vi "main OP700.vi"() -> ()   [LabVIEW 2020]
uses:
  SubVI/OP150ZP_state.ctl
  <userlib>/Alex.vi/FGV.ctl
  <vilib>/QMT/GDataBase for MySQL(tm)/MySQL/public/controls/DateType.ctl
  Lib/02 SLIM ZEN WS 500/SubVi/VG_progressBar.vi
  SubVI/CheminDeBase.vi
  <vilib>/Utility/error.llb/Error Cluster From Error Code.vi
  VG/PN.vi
  VG/IS30%.vi
  SubVI/VG_HYDRAU.vi
  VG/VG_BT3562.vi
  <vilib>/QMT/GDataBase for MySQL(tm)/MySQL/MySQLConnector.lvclass
panel:
  out "Revision":i32
  out "error out":errorcluster
  in  "arrêt":bool
  in  "last?":bool
  out "VISA OUT 2":T1
  out "Cluster 2":T2
  out "IS30% ?":bool
  out "BDD":T3
  out "progression":u8(slide) scale=0.0..100.0
  out "PN":string
  out "errout 2":errorcluster={"status"=TRUE, "code"=0, "source"="PCAN_CHANNEL ILLEGAL"} caption="errout"
  out "errout":errorcluster caption="sortie d'erreur"
  out "STOP":bool
  out "TOP":string
  out "DRAW":picture
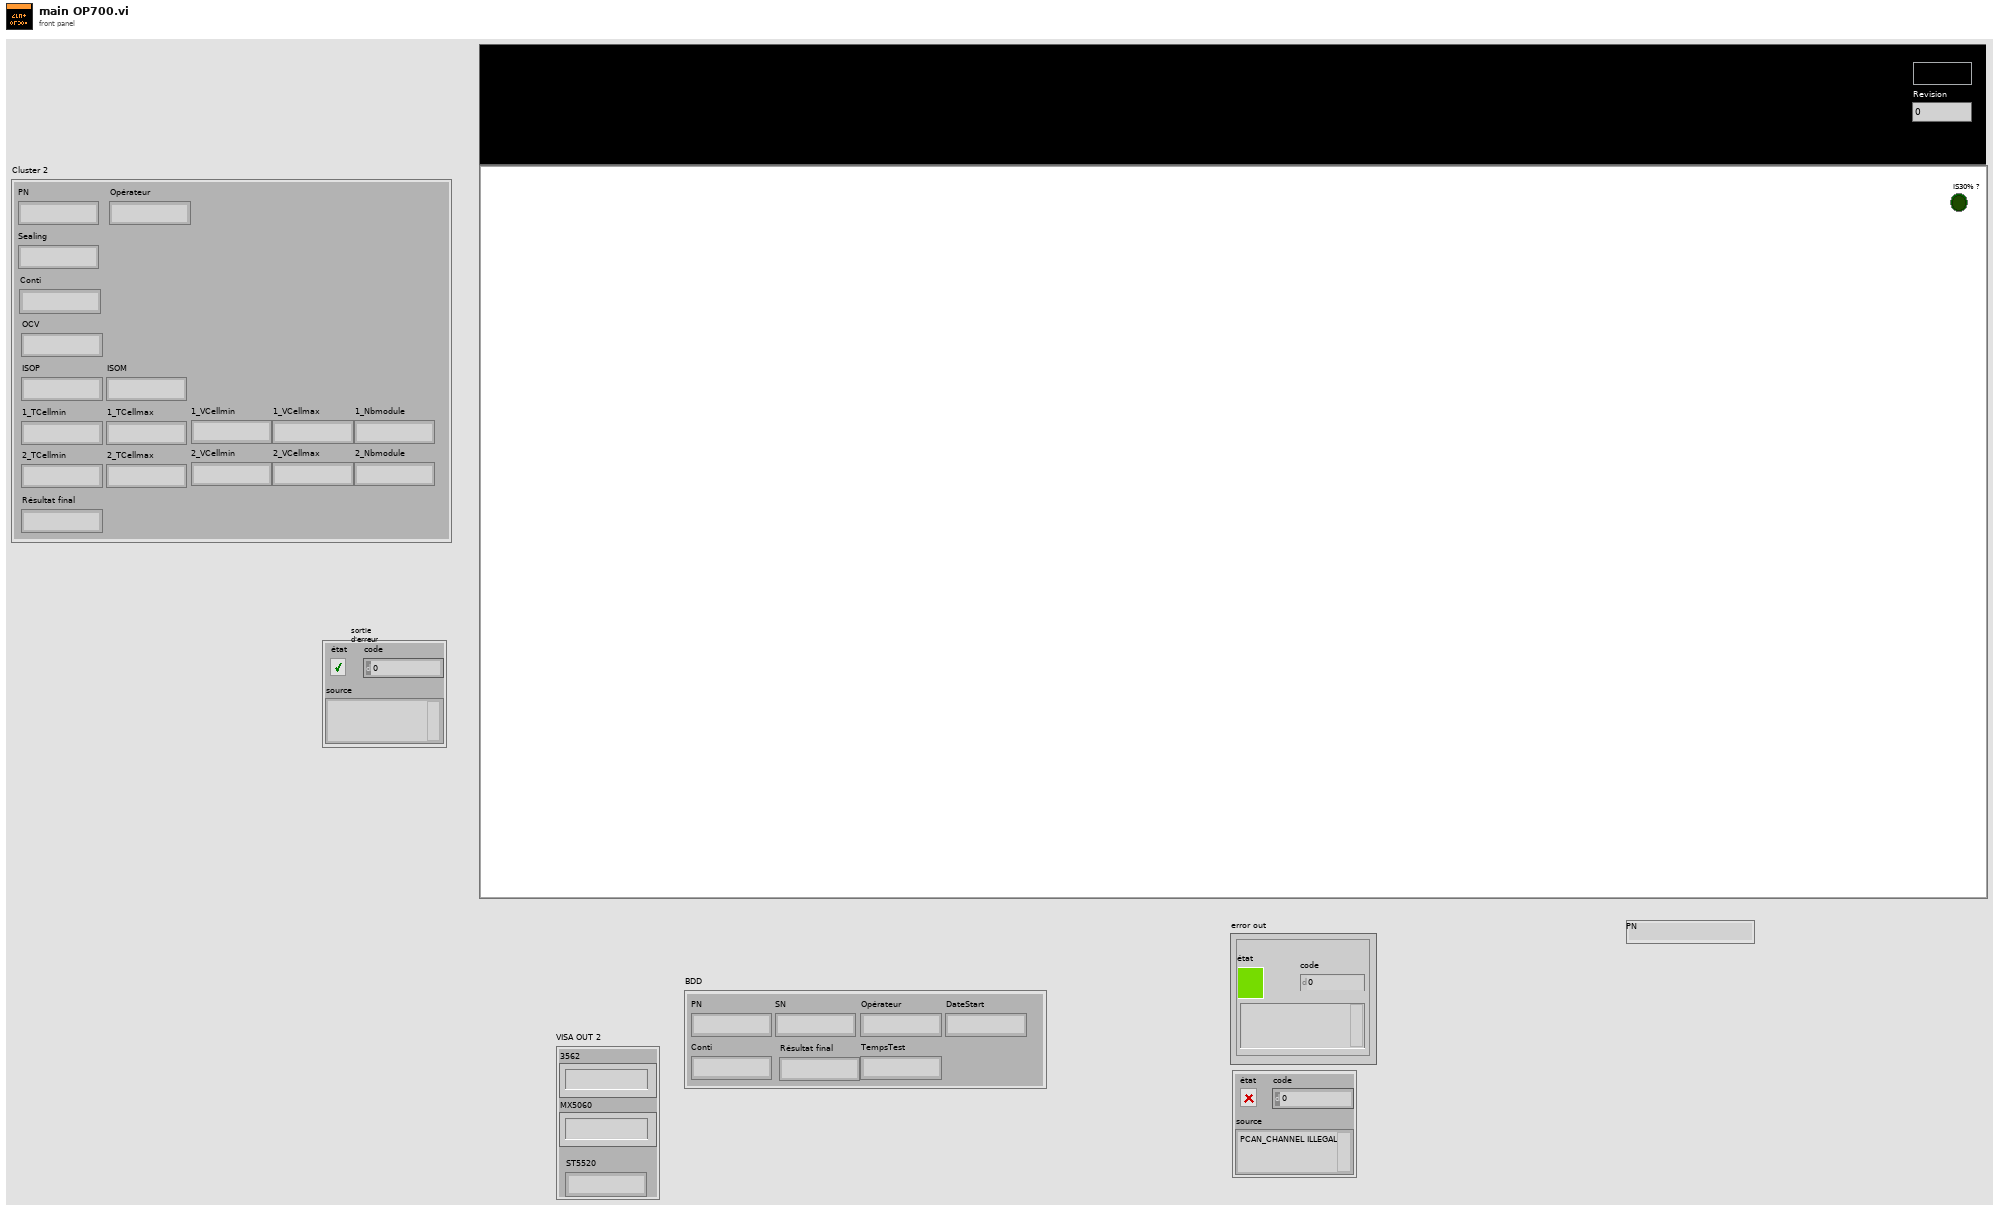
[diagram p1: front panel]
types:
  T1 = cluster{"3562":string, "MX5060":string, "ST5520":string}
  T2 = cluster{"PN":string, "Opérateur":string, "Sealing":string, "Conti":string, "OCV":string, "ISOP":string, "ISOM":string, "1_TCellmin":string, "1_TCellmax":string, "1_VCellmin":string, "1_VCellmax":string, "1_Nbmodule":string, "2_TCellmin":string, "2_TCellmax":string, "2_VCellmin":string, "2_VCellmax":string, "2_Nbmodule":string, "Résultat final":string}
  T3 = cluster{"PN":string, "Opérateur":string, "Conti":string, "Résultat final":string, "SN":string, "DateStart":string, "TempsTest":string}
  T4 = cluster{"PN":string, "Sealing":string, "Opérateur":string, "Conti":string, "OCV":string, "ISOP":string, "ISOP 2":string}
  T5 = typedef "OP150ZP_state.ctl" = enum16{"Null", "Demarrage", "Init", "Scan", "Crash", "Next", "Conti", "Sealing", "Comext", ""}
  T6 = typedef "FGV.ctl" = enum16{"GET", "SET", "RAZ"}
  T7 = typedef "MySQLVIEW.lvlib/MySQLConnector.lvclass/DateType.ctl" = enum16{"DATETIME", "DATE", "TIMESTAMP", "TIME", "YEAR (2 digits)", "YEAR (4 digits)"}
  T8 = typedef "imagedata.ctl" = cluster{"image type":i32, "image depth":i32, "image":u8[], "mask":u8[], "colors":u32[], "Rectangle":cluster{"left":i16, "top":i16, "right":i16, "bottom":i16}}
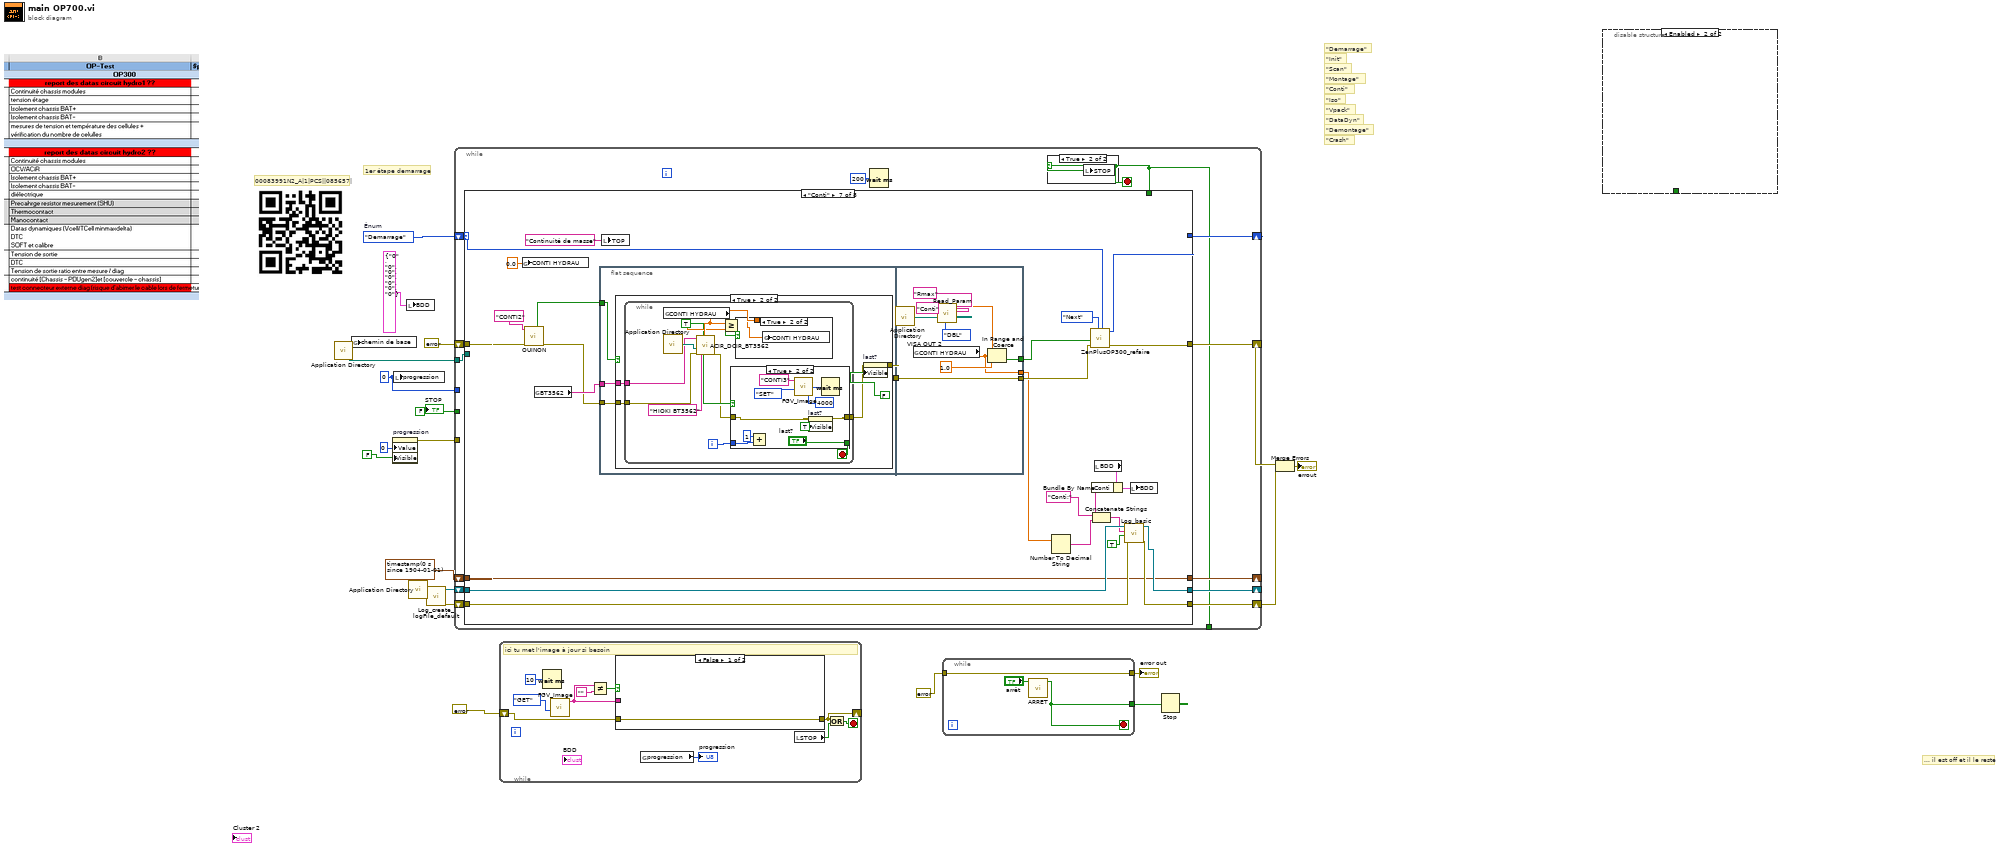
[diagram p0: block diagram]
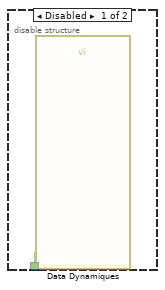
[diagram p2: hidden frame]
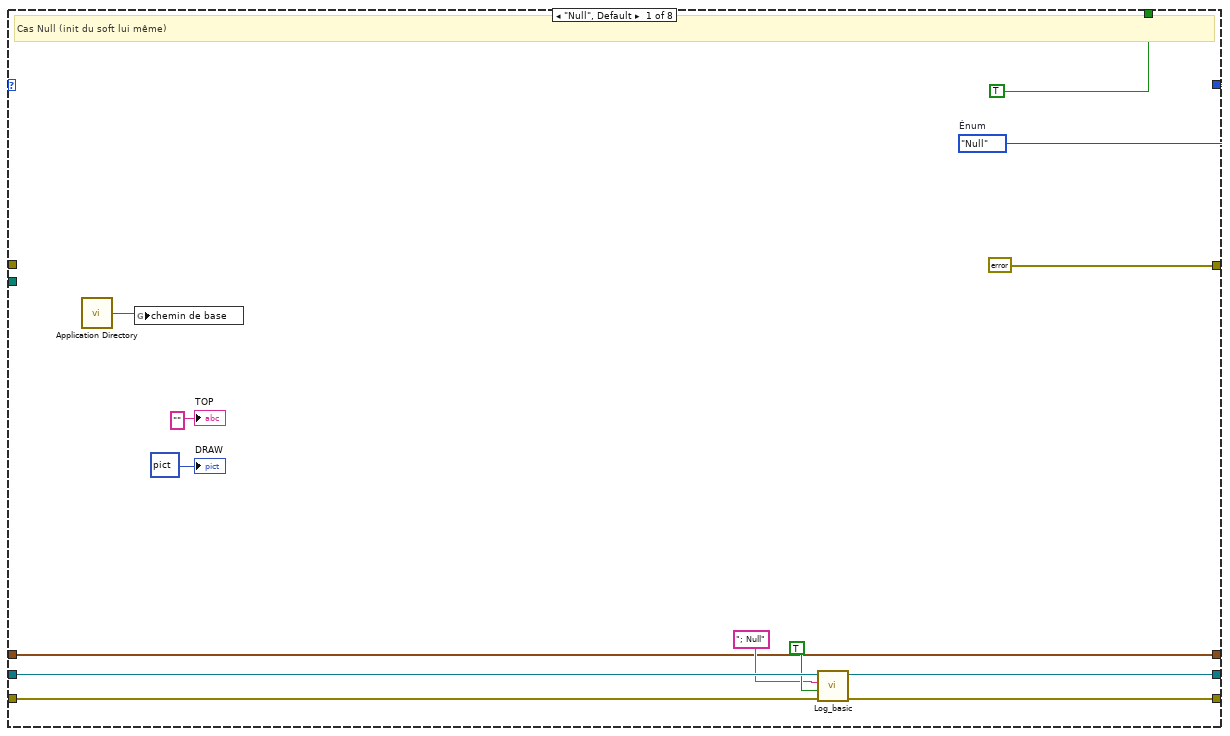
[diagram p4: hidden frame]
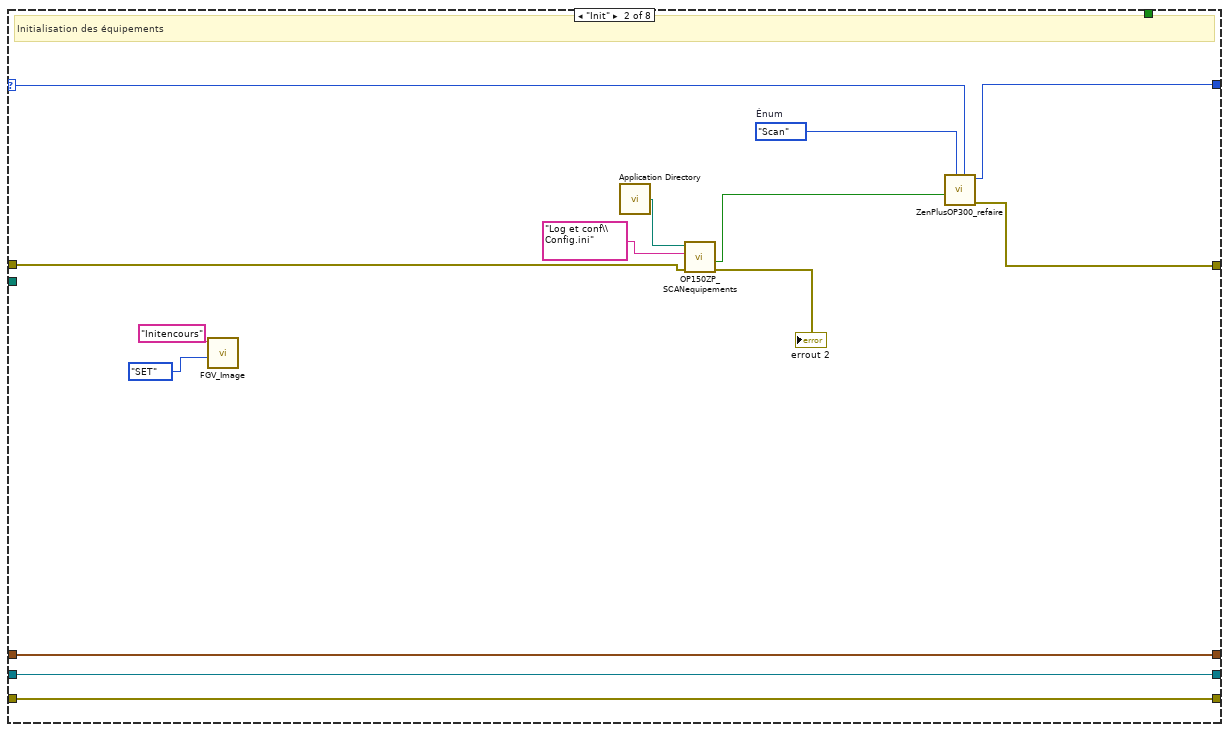
[diagram p5: hidden frame]
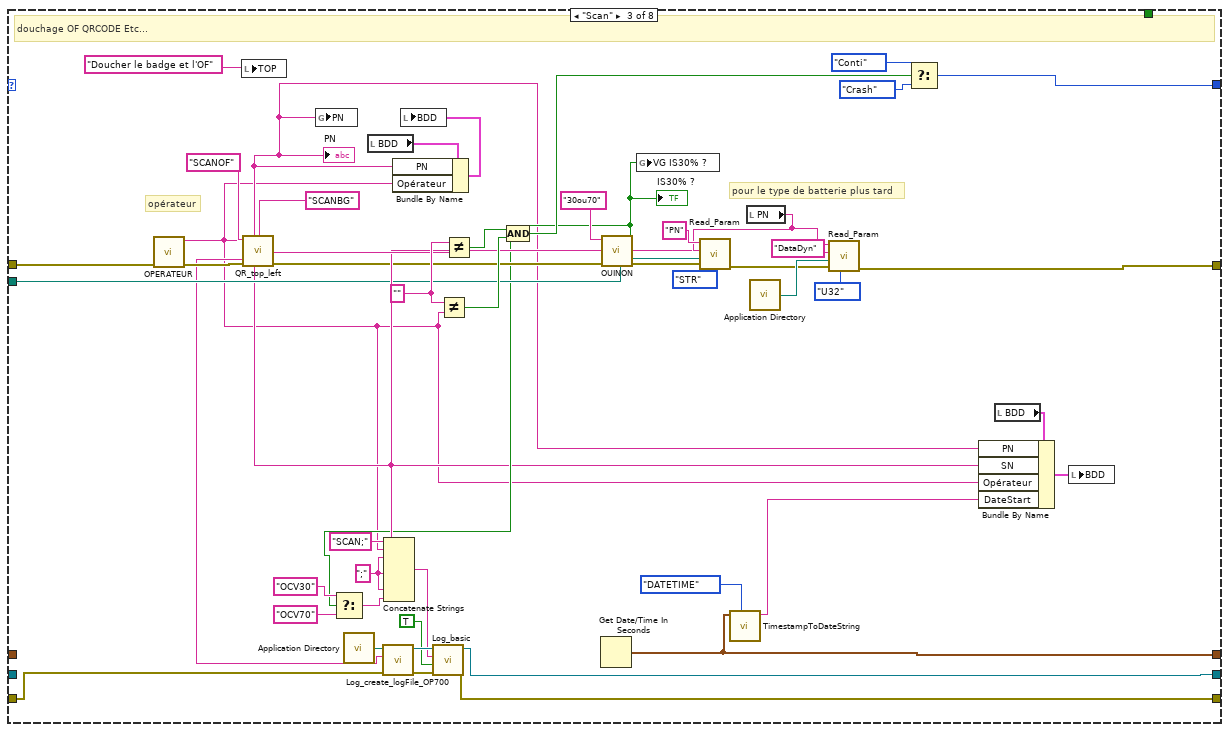
[diagram p6: hidden frame]
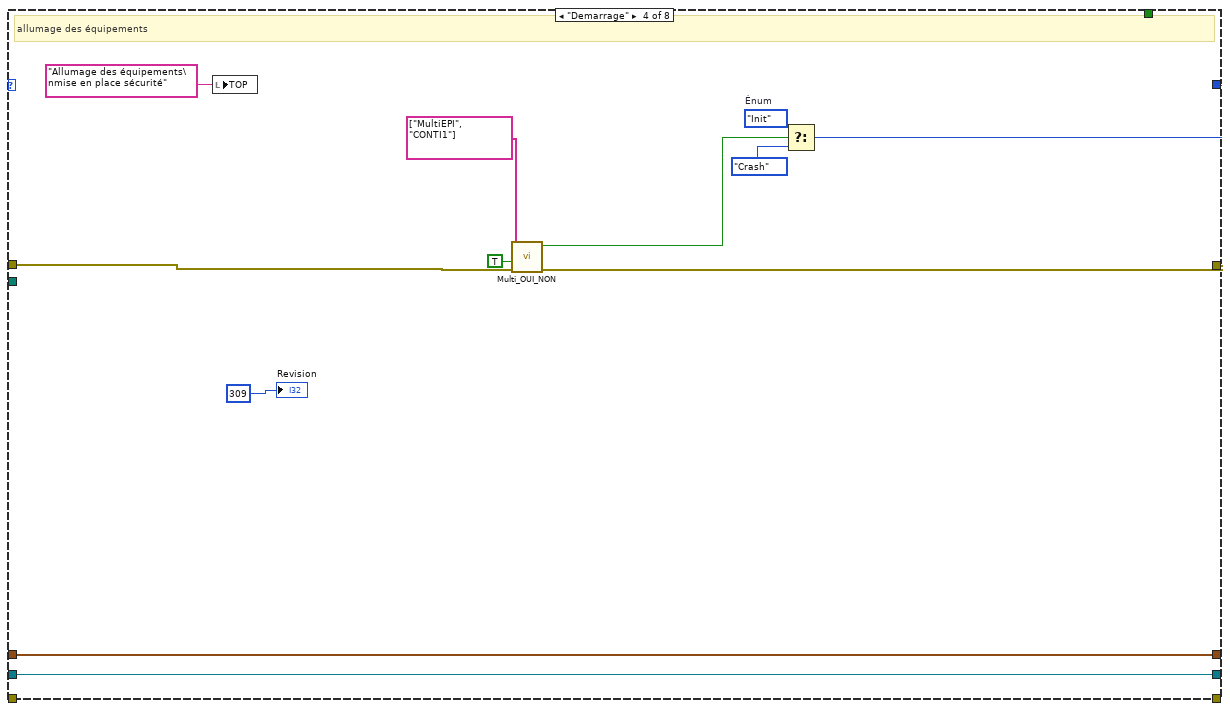
[diagram p7: hidden frame]
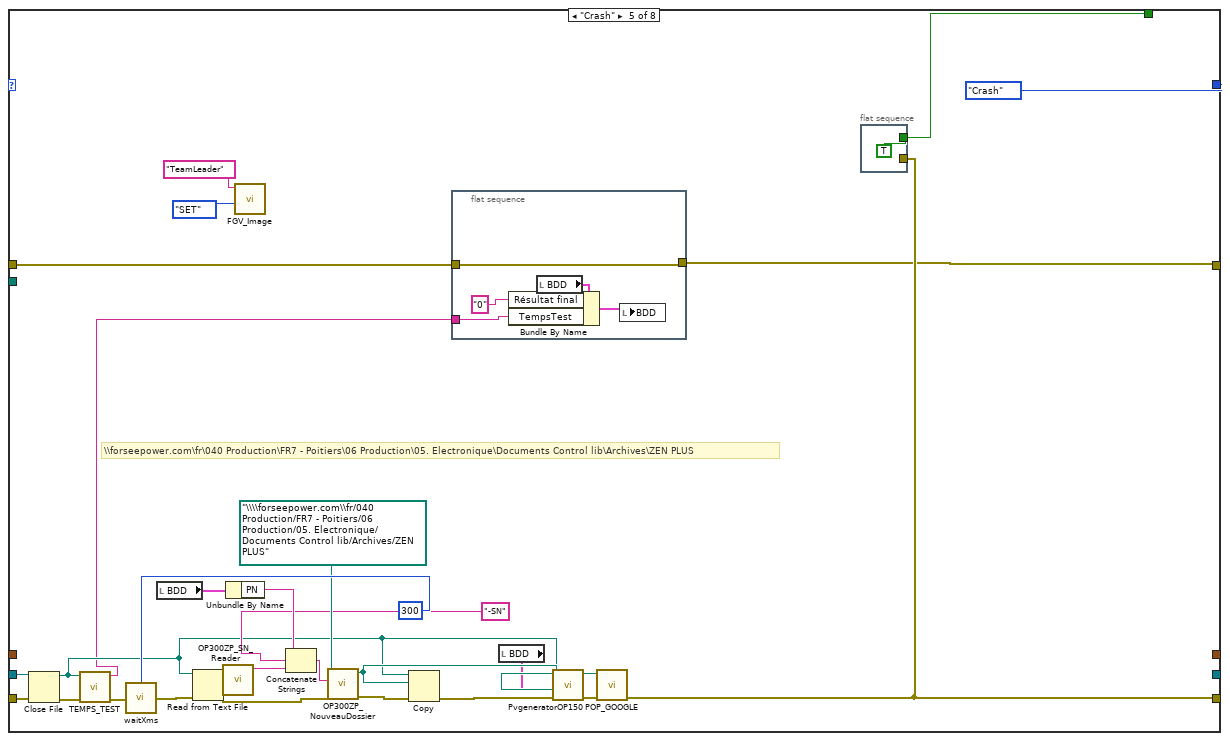
[diagram p8: hidden frame]
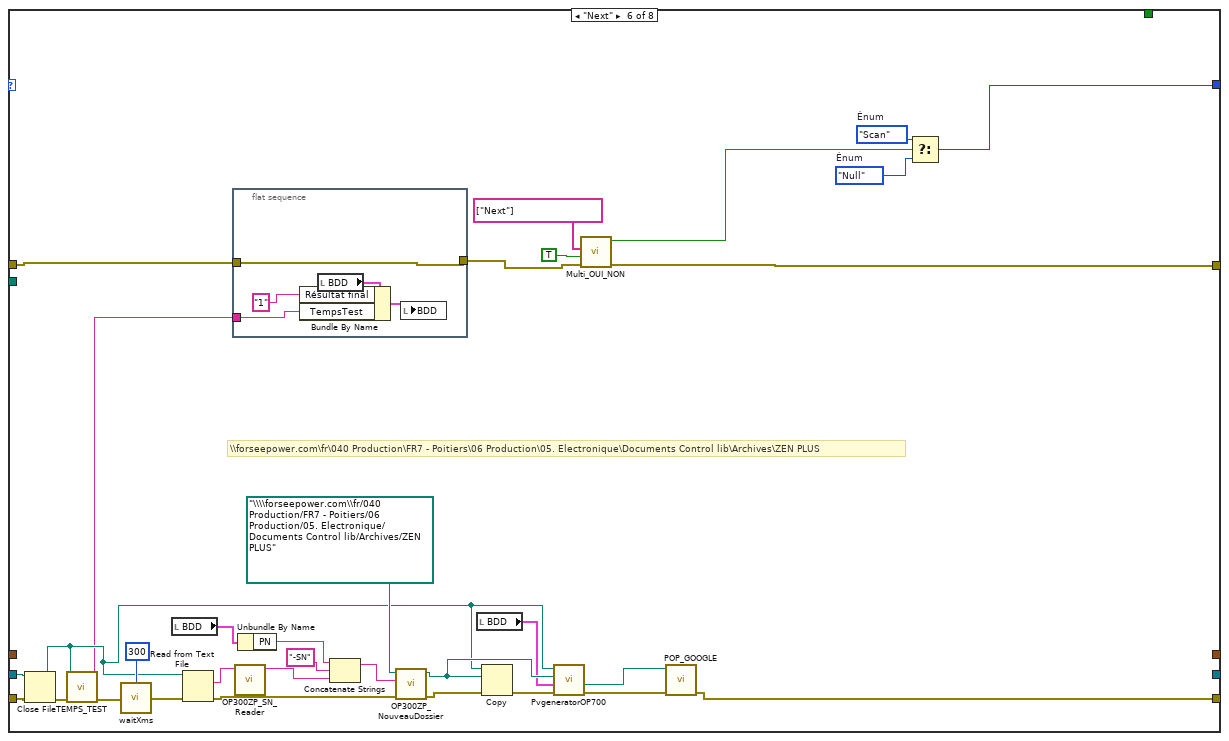
[diagram p9: hidden frame]
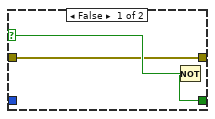
[diagram p11: hidden frame]
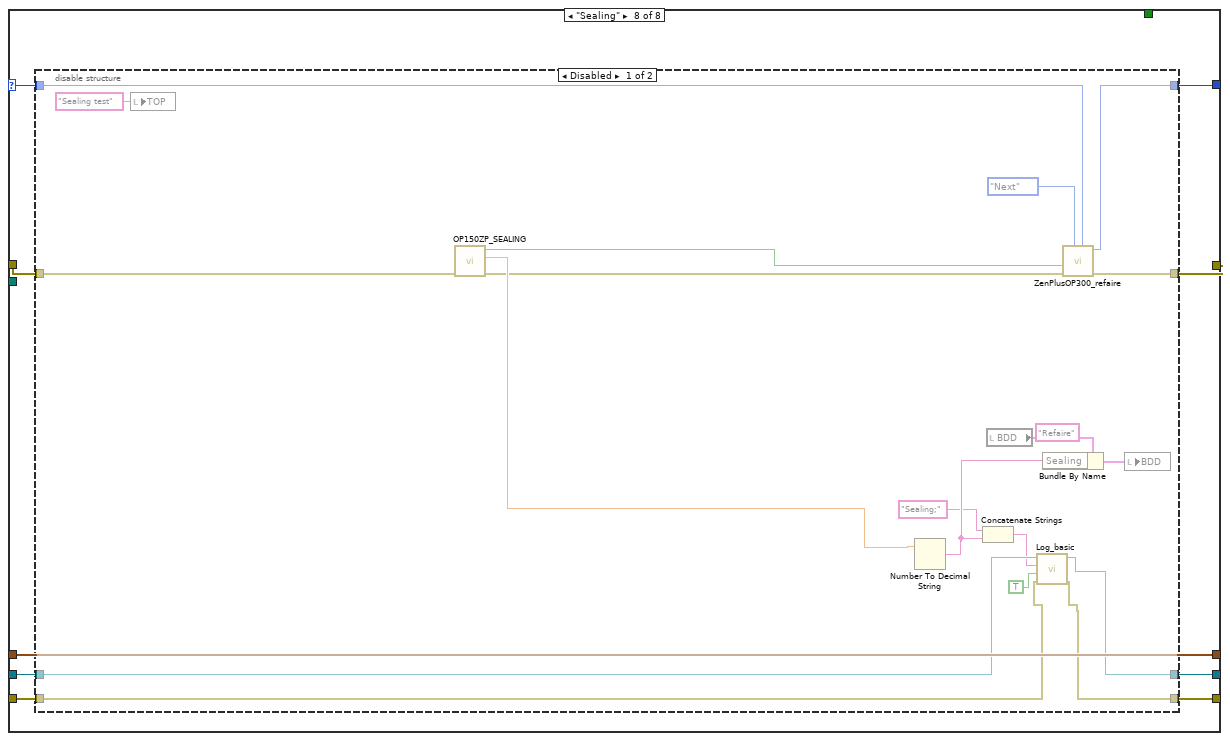
[diagram p13: hidden frame]
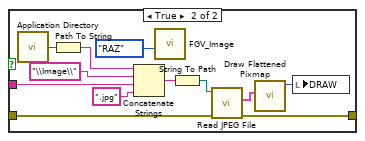
[diagram p15: hidden frame]
diagram:
  w10 = u8 0 ("progression")
  w11 = OP150ZP_state."Demarrage"  # Énum
  w17 = FALSE ("STOP")
  # "00083991N2_A|1|PCS||085657|"
  # "1er étape demarrage"
  # "\"Crash\""
  # "\"Demontage\""
  # "\"DataDyn\""
  # "\"Iso\""
  # "\"Montage\""
  # "\"Scan\""
  # "\"Init\""
  # "\"Demarrage\""
  # "\"Conti\""
  # "\"Vpack\""
  # "... il est off et il le reste"
  n1 = call <vilib>:"Application Directory.vi"() -> ("Application Directory"=w16:path)
  n2 = global write "CheminDeBase.vi" "chemin de base"(w16) -> ()
  n3 = property on="progression" class="Slide (strict)"("Value"=u8 0 ("progression"), "Visible"=FALSE) -> (error out=w8:errorcluster)  [unwired: 2 in, 1 out]
  n4 = local write "progression"(w10) -> ()
  n5 = local write "BDD"(T4 {"PN"="0", "Sealing"="0", "Opérateur"="0", "Conti"="0", "OCV"="0", "ISOP"="0", "ISOP 2"="0"} ("Cluster")) -> ()
  n6 = call <vilib>:"Application Directory.vi"() -> ("Application Directory"=w14:path)
  n7 = call "Log_create_logFile_default.vi"("appdir"=w14) -> ("errout"=w15:errorcluster, "Fichier à flux d'octets en sortie"=w18:refnum<file>)  [unwired: 9 in]
  n8 = while {
    shift-right: [w32] -> w3
    shift-left: errorcluster {"status"=FALSE, "code"=0, "source"=""} ("error out") -> [w23]
    shift-right: [w22] -> _
    shift-left: w11 -> [w27]
    shift-right: [w28] -> w19
    shift-left: w15 -> [w31]
    shift-right: [w29] -> _
    shift-left: w18 -> [w30]
    tunnel: w16 -> [w26]
    tunnel: w17 -> [_]
    shift-right: [w24] -> _
    shift-left: timestamp(0 s since 1904-01-01) ("seconds since 1Jan1904") -> [w25]
    tunnel: w10 -> [_]
    tunnel: w8 -> [_]
    tunnel: [w21] -> _
    stop <- w21 stop-if-true
    n9 = case shown="\"Conti\"" w27 {
      selector: w27 -> [_ w56 _ _ _ _ w220 w268]
      tunnel: w23 -> [_ w58 w111 w115 w129 w166 w221 w267]
      tunnel: [errorcluster {"status"=FALSE, "code"=0, "source"=""} ("errin") w57 w92 w122 w128 w170 w213 w272] -> w32
      tunnel: w31 -> [w43 w61 w107 _ w150 w189 w218 w275]
      tunnel: w30 -> [w44 w60 _ w123 w151 w190 w216 w274]
      tunnel: [w41 w60 w109 w123 _ _ w215 w273] -> w29
      tunnel: [w42 w61 w110 _ w142 w183 w217 w270] -> w28
      tunnel: [TRUE _ _ _ w152 _ _ _] -> w21
      tunnel: w26 -> [_ _ w86 _ _ _ _ _]
      tunnel: w25 -> [w37 w59 _ w121 _ _ w214 w271]
      tunnel: [w37 w59 w65 w121 _ _ w214 w271] -> w24
      tunnel: [w35 w48 w70 w116 OP150ZP_state."Crash" w167 w219 w269] -> w22
      frame "Null", Default {
        w35 = OP150ZP_state."Null"  # Énum
        # "Cas Null (init du soft lui même)"
        n10 = call <vilib>:"Application Directory.vi"() -> ("Application Directory"=w47:path)
        n11 = global write "CheminDeBase.vi" "chemin de base"(w47) -> ()
        n12 = call "Log_basic.vi"("errin"=w43, "date?"=TRUE, "chaîne"="; Null", "in"=w44) -> ("sortie d'erreur"=w42:errorcluster, "refnum en sortie"=w41:refnum<file>)  [unwired: 6 in]
        "DRAW" <- picture data[5B] ("DRAW")
        "TOP" <- "" ("TOP")
      }
      frame "Init" {
        w52 = OP150ZP_state."Scan"  # Énum
        # "Initialisation des équipements"
        n13 = call <userlib>:"FGV_Image.vi"("Énum"=FGV."SET", "IN"="Initencours") -> ()  [unwired: 9 in, 1 out]
        n14 = call <vilib>:"Application Directory.vi"() -> ("Application Directory"=w49:path)
        n15 = call "OP150ZP_SCANequipements.vi"("Errin"=w58, "Chaîne"="Log et conf\\Config.ini", "pathin"=w49) -> ("ERROUT"=→"errout 2":errorcluster, "KO?"=w53:bool)  [unwired: 7 in]
        n16 = call "ZenPlusOP300_refaire.vi"("refaire"=w56, "casOK"=w52, "test ok ?"=w53) -> ("errout"=w57:errorcluster, "Next"=w48:T5)  [unwired: 7 in]
      }
      frame "Scan" {
        w73 = ";" ("chaîne")
        w101 = "" ("x")
        # "pour le type de batterie plus tard"
        # "opérateur"
        # "douchage OF QRCODE Etc..."
        n17 = call "OPERATEUR.vi"("errin"=w111, "IN"="SCANBG") -> ("error out"=w98:errorcluster, "Dataout"=w66:string)  [unwired: 8 in]
        n18 = local write "TOP"("Doucher le badge et l'OF" ("TOP")) -> ()
        n19 = call "QR_top_left.vi"("errin"=w98, "image"="SCANOF") -> ("error out"=w77:errorcluster, "Réponse"=w96:string, "SN"=w67:string, "PN"=w68:string)  [unwired: 5 in, 1 out]
        "PN" <- w68
        n20 = global write "PN.vi" "PN"(w68) -> ()
        n21 = call <vilib>:"Application Directory.vi"() -> ("Application Directory"=w108:path)
        n22 = local read "BDD"() -> (w80:T3)
        n23 = call "Log_create_logFile_OP700.vi"("errin"=w107, "toute l'expression"=w67, "Application Directory"=w108) -> ("sortie d'erreur"=w105:errorcluster, "Fichier à flux d'octets en sortie"=w106:refnum<file>)  [unwired: 7 in]
        n24 = Bundle By Name(cluster=w80, "PN"=w68, "Opérateur"=w66) -> (w79:T3)
        n25 = local write "BDD"(w79) -> ()
        n26 = Not Equal?(x=w101, y=w66) -> (x != y?=w99:bool)
        n27 = Not Equal?(x=w101, y=w96) -> (x != y?=w100:bool)
        n28 = Compound Arithmetic op=AND ("Opérateur arithmétique")(w100, w99) -> (w84:bool)
        n29 = Get Date/Time In Seconds() -> (seconds since 1Jan1904=w65:timestamp)
        n30 = call "OUINON.vi"("errin"=w77, "image"="30ou70") -> ("error out"=w76:errorcluster, "OUI/NON"=w71:bool)  [unwired: 8 in]
        "IS30% ?" <- w71
        n31 = Select ("Sélectionner")(t="OCV30" ("section"), s=w71, f="OCV70" ("section")) -> (s? t:f=w72:string)
        n32 = global write "IS30%.vi" "VG IS30% ?"(w71) -> ()
        n33 = call <vilib>:"TimestampToDateString.vi"("dateType"=DateType."DATETIME", "timestamp in"=w65) -> ("dateString"=w64:string)  [unwired: 8 in, 1 out]
        n34 = local read "PN"() -> (w88:string)
        n35 = call "Read_Param.vi"("Énum"=enum16{"STR", "DBL", "U32"}."STR", "errin"=w76, "pathin"=w86, "section"=w88, "key"="PN") -> ("error out"=w91:errorcluster, "str"=w87:string)  [unwired: 2 in, 3 out]
        n36 = Concatenate Strings("SCAN;" ("chaîne"), w66, w73, w67, w73, w87, w73, w72) -> (w103:string)
        n37 = call "Log_basic.vi"("errin"=w105, "date?"=TRUE, "chaîne"=w103, "in"=w106) -> ("sortie d'erreur"=w110:errorcluster, "refnum en sortie"=w109:refnum<file>)  [unwired: 6 in]
        n38 = call <vilib>:"Application Directory.vi"() -> ("Application Directory"=w95:path)
        n39 = call "Read_Param.vi"("Énum"=enum16{"STR", "DBL", "U32"}."U32", "errin"=w91, "pathin"=w95, "section"="DataDyn", "key"=w88) -> ("error out"=w92:errorcluster)  [unwired: 2 in, 4 out]
        n40 = Select ("Sélectionner")(t=OP150ZP_state."Conti" ("Énum"), s=w84, f=OP150ZP_state."Crash" ("cas faux")) -> (s? t:f=w70:T5)
        n41 = local read "BDD"() -> (w69:T3)
        n42 = Bundle By Name(cluster=w69, "PN"=w68, "SN"=w67, "Opérateur"=w66, "DateStart"=w64) -> (w63:T3)
        n43 = local write "BDD"(w63) -> ()
      }
      frame "Demarrage" {
        w118 = OP150ZP_state."Init"  # Énum
        # "allumage des équipements"
        n44 = local write "TOP"("Allumage des équipements\nmise en place sécurité" ("TOP")) -> ()
        n45 = call "Multi_OUI_NON.vi"("errin"=w115, "errinb"=TRUE, "Tableau"=string[] ["MultiEPI", "CONTI1"]) -> ("errout"=w122:errorcluster, "isok?"=w119:bool)  [unwired: 7 in]
        n46 = Select ("Sélectionner")(t=w118, s=w119, f=OP150ZP_state."Crash" ("cas faux")) -> (s? t:f=w116:T5)
        "Revision" <- 309
      }
      frame "Crash" {
        # "\\\\forseepower.com\\fr\\040 Production\\FR7 - Poitiers\\06 Production\\05. Electronique\\Documents Control lib\\Archives\\ZEN PLUS"
        n47 = Close File(refnum=w151, error in=w150) -> (path=w126:path, error out=w144:errorcluster)
        n48 = call <userlib>:"TEMPS_TEST.vi"("errin"=w144, "pathin"=w126) -> ("error out"=w127:errorcluster, "Delay calculé"=w125:string)  [unwired: 8 in]
        n49 = call <userlib>:"waitXms.vi"("attente (ms)"=u32 300, "errin"=w127) -> ("errout"=w141:errorcluster)  [unwired: 13 in]
        n50 = local read "BDD"() -> (w135:T3)
        n51 = Read from Text File(file (use dialog)=w126, error in=w141) -> (text=w140:string, error out=w138:errorcluster)  [unwired: 2 in, 2 out]
        n52 = call "OP300ZP_SN_Reader.vi"("Fichier txt"=w140) -> ("SN"=w133:string)  [unwired: 10 in]
        n53 = Unbundle By Name(w135) -> ("PN"=w132:string)
        n54 = call <userlib>:"FGV_Image.vi"("Énum"=FGV."SET", "IN"="TeamLeader") -> ()  [unwired: 9 in, 1 out]
        n55 = Concatenate Strings(w132, "-SN" ("chaîne"), w133) -> (w134:string)
        n56 = call "OP300ZP_NouveauDossier.vi"("entrée d'erreur (pas d'erreur)"=w138, "Nom du repertoire (PN SN)"=w134, "Network before adding a new folder"=path "\\\\forseepower.com\\fr/040 Production/FR7 - Poitiers/06 Production/05. Electronique/Documents Control lib/Archives/ZEN PLUS" ("chemin de la cible (utiliser une boîte de dialogue)")) -> ("sortie d'erreur"=w139:errorcluster, "Network after adding a new folder"=w136:path)  [unwired: 7 in]
        n57 = Copy ("Copier")(8:w139, 10:w136, 11:w126) -> (0:w143:errorcluster)  [unwired: 2 in, 2 out]
        n58 = flat-sequence {
          tunnel: [w155] -> w128
          tunnel: w129 -> [w155]
          tunnel: w125 -> [w153]
          frame #0 {
            n59 = local read "BDD"() -> (w157:T3)
            n60 = Bundle By Name(cluster=w157, "Résultat final"="0", "TempsTest"=w153) -> (w154:T3)
            n61 = local write "BDD"(w154) -> ()
          }
        }
        n62 = local read "BDD"() -> (w124:T3)
        n63 = call "PvgeneratorOP150.vi"("errin"=w143, "BDD"=w124, "network"=w136, "path in"=w126) -> ("sortie d'erreur"=w147:errorcluster, "network out"=w146:path)  [unwired: 4 in, 2 out]
        n64 = call "POP_GOOGLE.vi"("error in"=w147, "chemin"=w146) -> ("error out"=w142:errorcluster)  [unwired: 8 in, 1 out]
        n65 = flat-sequence {
          tunnel: [TRUE] -> w152
          tunnel: w142 -> [_]
          frame #0 {
          }
        }
      }
      frame "Next" {
        w187 = OP150ZP_state."Null"  # Énum
        w188 = OP150ZP_state."Scan"  # Énum
        # "\\\\forseepower.com\\fr\\040 Production\\FR7 - Poitiers\\06 Production\\05. Electronique\\Documents Control lib\\Archives\\ZEN PLUS"
        n66 = Close File(refnum=w190, error in=w189) -> (path=w163:path, error out=w164:errorcluster)
        n67 = call <userlib>:"TEMPS_TEST.vi"("errin"=w164, "pathin"=w163) -> ("error out"=w161:errorcluster, "Delay calculé"=w160:string)  [unwired: 8 in]
        n68 = call <userlib>:"waitXms.vi"("attente (ms)"=u32 300, "errin"=w161) -> ("errout"=w162:errorcluster)  [unwired: 13 in]
        n69 = local read "BDD"() -> (w176:T3)
        n70 = Read from Text File(file (use dialog)=w163, error in=w162) -> (text=w181:string, error out=w180:errorcluster)  [unwired: 2 in, 2 out]
        n71 = flat-sequence {
          tunnel: [w193] -> w165
          tunnel: w166 -> [w193]
          tunnel: w160 -> [w191]
          frame #0 {
            n72 = local read "BDD"() -> (w195:T3)
            n73 = Bundle By Name(cluster=w195, "Résultat final"="1", "TempsTest"=w191) -> (w192:T3)
            n74 = local write "BDD"(w192) -> ()
          }
        }
        n75 = call "OP300ZP_SN_Reader.vi"("Fichier txt"=w181) -> ("SN"=w173:string)  [unwired: 10 in]
        n76 = Unbundle By Name(w176) -> ("PN"=w175:string)
        n77 = Concatenate Strings(w175, "-SN" ("chaîne"), w173) -> (w172:string)
        n78 = call "OP300ZP_NouveauDossier.vi"("entrée d'erreur (pas d'erreur)"=w180, "Nom du repertoire (PN SN)"=w172, "Network before adding a new folder"=path "\\\\forseepower.com\\fr/040 Production/FR7 - Poitiers/06 Production/05. Electronique/Documents Control lib/Archives/ZEN PLUS" ("chemin de la cible (utiliser une boîte de dialogue)")) -> ("sortie d'erreur"=w179:errorcluster, "Network after adding a new folder"=w177:path)  [unwired: 7 in]
        n79 = local read "BDD"() -> (w159:T3)
        n80 = Copy ("Copier")(8:w179, 10:w177, 11:w163) -> (0:w182:errorcluster)  [unwired: 2 in, 2 out]
        n81 = call "PvgeneratorOP700.vi"("errin"=w182, "BDD"=w159, "network"=w177, "path in"=w163) -> ("sortie d'erreur"=w185:errorcluster, "network out"=w184:path)  [unwired: 4 in, 2 out]
        n82 = call "Multi_OUI_NON.vi"("errin"=w165, "errinb"=TRUE, "Tableau"=string[] ["Next"]) -> ("errout"=w170:errorcluster, "isok?"=w169:bool)  [unwired: 7 in]
        n83 = call "POP_GOOGLE.vi"("error in"=w185, "chemin"=w184) -> ("error out"=w183:errorcluster)  [unwired: 8 in, 1 out]
        n84 = Select(t=w188, s=w169, f=w187) -> (s? t:f=w167:T5)
      }
      frame "Conti" {
        n85 = global write "VG_HYDRAU.vi" "CONTI HYDRAU"(0.0 ("R")) -> ()
        n86 = call "OUINON.vi"("errin"=w221, "image"="CONTI2" ("IN")) -> ("error out"=w196:errorcluster, "OUI/NON"=w208:bool)  [unwired: 8 in]
        n87 = global read "VG_BT3562.vi" "BT3562"() -> (w203:string)
        n88 = flat-sequence {
          tunnel: w208 -> [w225]
          tunnel: w203 -> [w224]
          tunnel: [w223] -> w212
          tunnel: w196 -> [w222]
          tunnel: [w260] -> w204
          tunnel: [w259] -> w205
          tunnel: [w258] -> w206
          tunnel: w212 -> [w258]
          frame #0 {
            n89 = case shown="True" w225 {
              tunnel: w224 -> [_ w231]
              tunnel: [w226 w229] -> w223
              tunnel: w222 -> [w226 w227]
              frame False {
              }
              frame True {
                n90 = while {
                  tunnel: w231 -> [w235]
                  tunnel: [w242] -> w228
                  tunnel: w227 -> [w233]
                  i -> [w241]
                  stop <- w238 stop-if-true
                  n91 = global read "VG_HYDRAU.vi" "CONTI HYDRAU"() -> (w236:dbl)
                  n92 = call <vilib>:"Application Directory.vi"() -> ("Application Directory"=w244:path)
                  n93 = call <userlib>:"ACIR_DCIR_BT3562.vi"("juste R?"=TRUE, "errin"=w233, "chemin de base"=w244, "section"="HIOKI BT3562", "VISAin"=w235) -> ("errout"=w237:errorcluster, "OK?"=w243:bool, "R"=w239:dbl)  [unwired: 4 out]
                  n94 = Greater Or Equal?(x=w239, y=w236) -> (x >= y?=w240:bool)
                  n95 = case shown="True" w243 {
                    selector: w243 -> [w247 _]
                    tunnel: w237 -> [w245 w249]
                    tunnel: [w245 w251] -> w242
                    tunnel: [w246 "last?"] -> w238
                    tunnel: w241 -> [_ w254]
                    frame False {
                      n96 = Not(x=w247) -> (.not. x?=w246:bool)
                    }
                    frame True {
                      n97 = Add(x=1, y=w254) -> ()  [unwired: 1 out]
                      n98 = call <userlib>:"FGV_Image.vi"("Énum"=FGV."SET", "IN"="CONTI3") -> ()  [unwired: 9 in, 1 out]
                      n99 = property on="last?" class="Bool"(error in=w249, "Visible"=TRUE) -> (error out=w251:errorcluster)  [unwired: 1 in, 1 out]
                      n100 = Wait (ms)(milliseconds to wait=u32 4000 ("attente (ms)")) -> ()  [unwired: 1 out]
                    }
                  }
                  n101 = case shown="True" w240 {
                    tunnel: w239 -> [_ w257]
                    frame False {
                    }
                    frame True {
                      n102 = global write "VG_HYDRAU.vi" "CONTI HYDRAU"(w257) -> ()
                    }
                  }
                }
                n103 = property on="last?" class="Bool"(error in=w228, "Visible"=FALSE) -> (error out=w229:errorcluster)  [unwired: 1 in, 1 out]
              }
            }
          }
          frame #1 {
            n104 = call <vilib>:"Application Directory.vi"() -> ("Application Directory"=w264:path)
            n105 = global read "VG_HYDRAU.vi" "CONTI HYDRAU"() -> (w259:dbl)
            n106 = call "Read_Param.vi"("Énum"=enum16{"STR", "DBL", "U32"}."DBL", "pathin"=w264, "section"="Conti", "key"="Rmax") -> ("dbl"=w262:dbl)  [unwired: 3 in, 4 out]
            n107 = In Range and Coerce(upper limit=w262, x=w259, lower limit=1.0 ("limite inférieure")) -> (In Range?=w260:bool)  [unwired: 1 out]
          }
        }
        n108 = local write "TOP"("Continuité de masse" ("TOP")) -> ()
        n109 = Number To Decimal String(number=w205) -> (decimal integer string=w200:string)  [unwired: 1 in]
        n110 = call "ZenPlusOP300_refaire.vi"("refaire"=w220, "casOK"=OP150ZP_state."Next" ("refaire"), "errin"=w206, "test ok ?"=w204) -> ("errout"=w213:errorcluster, "Next"=w219:T5)  [unwired: 6 in]
        n111 = Concatenate Strings("Conti;" ("chaîne"), w200) -> (w198:string)
        n112 = local read "BDD"() -> (w201:T3)
        n113 = Bundle By Name(cluster=w201, "Conti"=w200) -> (w202:T3)
        n114 = call "Log_basic.vi"("errin"=w218, "date?"=TRUE, "chaîne"=w198, "in"=w216) -> ("sortie d'erreur"=w217:errorcluster, "refnum en sortie"=w215:refnum<file>)  [unwired: 6 in]
        n115 = local write "BDD"(w202) -> ()
      }
      frame "Sealing" {
        n116 = disable-structure shown="Disabled" {
          disable-tunnel: w275 -> [w294 _]
          disable-tunnel: w274 -> [w293 _]
          disable-tunnel: [w292 _] -> w273
          disable-tunnel: [w291 _] -> w272
          disable-tunnel: [w287 _] -> w270
          disable-tunnel: [w286 _] -> w269
          disable-tunnel: w268 -> [w284 _]
          disable-tunnel: w267 -> [w282 _]
          frame Disabled {
            (unwired) "Refaire" ("image")
            n117 = local write "TOP"("Sealing test" ("TOP")) -> ()
            n118 = call "OP150ZP_SEALING.vi"("ERRIN"=w282) -> ("ERROUT"=w276:errorcluster, "SEALING_VALUE"=w281:dbl, "IsOK?"=w277:bool)  [unwired: 8 in]
            n119 = Number To Decimal String(number=w281) -> (decimal integer string=w288:string)  [unwired: 1 in]
            n120 = Concatenate Strings("Sealing;" ("chaîne"), w288) -> (w279:string)
            n121 = local read "BDD"() -> (w290:T3)
            n122 = call "Log_basic.vi"("errin"=w294, "date?"=TRUE, "chaîne"=w279, "in"=w293) -> ("sortie d'erreur"=w287:errorcluster, "refnum en sortie"=w292:refnum<file>)  [unwired: 6 in]
            n123 = Bundle By Name(cluster=w290, "Sealing"=w288) -> (w289:T3)
            n124 = call "ZenPlusOP300_refaire.vi"("refaire"=w284, "casOK"=OP150ZP_state."Next" ("refaire"), "errin"=w276, "test ok ?"=w277) -> ("errout"=w291:errorcluster, "Next"=w286:T5)  [unwired: 6 in]
            n125 = local write "BDD"(w289) -> ()
          }
          frame Enabled {
          }
        }
      }
    }
    n126 = Wait (ms)(milliseconds to wait=u32 200 ("attente (ms)")) -> ()  [unwired: 1 out]
    n127 = case shown="True" w21 {
      selector: w21 -> [_ w34]
      frame False {
      }
      frame True {
        n128 = local write "STOP"(w34) -> ()
      }
    }
  }
  n129 = while {
    shift-right: [w303] -> _
    shift-left: errorcluster {"status"=FALSE, "code"=0, "source"=""} ("error out") -> [w300]
    stop <- w301 stop-if-true
    # "ici tu met l'image à jour si besoin"
    n130 = Wait (ms)(milliseconds to wait=u32 10 ("attente (ms)")) -> ()  [unwired: 1 out]
    n131 = call <userlib>:"FGV_Image.vi"("Énum"=FGV."GET") -> ("OUT"=w296:string)  [unwired: 10 in]
    n132 = Not Equal?(x=w296, y="") -> (x != y?=w297:bool)
    n133 = case shown="False" w297 {
      tunnel: [w305 w310] -> w303
      tunnel: w300 -> [w305 w309]
      tunnel: w296 -> [_ w308]
      frame False {
      }
      frame True {
        n134 = call <vilib>:"Application Directory.vi"() -> ("Application Directory"=w313:path)
        n135 = Path To String(path=w313) -> (string=w314:string)
        n136 = Concatenate Strings(w314, "\\Image\\" ("chaîne"), w308, ".jpg" ("chaîne")) -> (w312:string)
        n137 = call <userlib>:"FGV_Image.vi"("Énum"=FGV."RAZ") -> ()  [unwired: 10 in, 1 out]
        n138 = String To Path(string=w312) -> (path=w311:path)
        n139 = call <vilib>:"Read JPEG File.vi"("error in (no error)"=w309, "path to JPEG file"=w311) -> ("error out"=w310:errorcluster, "image data"=w317:T8)  [unwired: 7 in, 1 out]
        n140 = call <vilib>:"Draw Flattened Pixmap.vi"("image data"=w317) -> ("new picture"=w306:picture)  [unwired: 8 in]
        n141 = local write "DRAW"(w306) -> ()
      }
    }
    n142 = global read "VG_progressBar.vi" "progression"() -> (→"progression":u8)
    n143 = local read "STOP"() -> (w302:bool)
    n144 = Or(x=w303, y=w302) -> (x .or. y?=w301:bool)
  }
  n145 = while {
    tunnel: [w319] -> w4
    tunnel: errorcluster {"status"=FALSE, "code"=0, "source"=""} ("error out") -> [w319]
    tunnel: [w318] -> w2
    stop <- w318 stop-if-true
    n146 = call <userlib>:"ARRET.vi"("arrêt"="arrêt") -> ("T button?"=w318:bool)  [unwired: 10 in]
  }
  "error out" <- w4
  n147 = Stop(stop? (T)=w2) -> ()
  n148 = Merge Errors(w3, w19) -> (→"errout":errorcluster)
  n149 = disable-structure shown="Enabled" {
    disable-tunnel: [w321 _] -> _
    frame Disabled {
      n150 = call "Data Dynamiques"() -> ("CMU OK"=w321:bool)  [unwired: 12 in, 7 out]
    }
    frame Enabled {
    }
  }
  "STOP" <- w17
